vi "Get Named Tag Data.vi"(8 "error in (no error)":errorcluster, 10 "Tag Name":string, 11 "Raw Message in":refnum<class "Raw Message.lvclass">) -> (0 "error out":errorcluster, 1 "Tag Data":variant[](array[variant]), 2 "Key not found?":bool, 3 "Raw Message out":refnum<class "Raw Message.lvclass">)   [LabVIEW 2020]
uses:
  Raw Message.lvclass/Raw Message.ctl
  Tag/Basic Type.lvclass
  Raw Message.lvclass
  E:/Labview/LV 2020/Libs/LV Protobuf Raw/Source/Tag/Basic Type.lvclass
  E:/Labview/LV 2020/Libs/LV Protobuf Raw/Source/Proto Value/Proto Type.lvclass
  E:/Labview/LV 2020/Libs/LV Protobuf Raw/Source/Type Serializer/Type Serializer.lvclass
  E:/Labview/LV 2020/Libs/LV Protobuf Raw/Source/String Representable/String Representable.lvclass
  E:/Labview/LV 2020/Libs/LV Protobuf Raw/Source/Wire Type Group/Wire Type Group.lvclass
  E:/Labview/LV 2020/Libs/LV Protobuf Raw/Source/LEN Encoder/LEN.lvclass
  E:/Labview/LV 2020/Libs/LV Protobuf Raw/Source/Message/Raw Message.lvclass
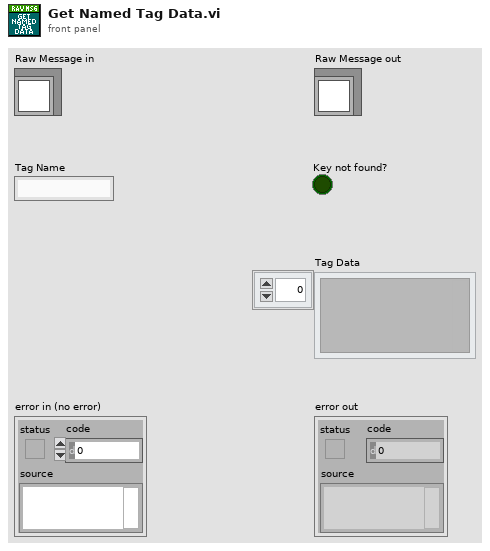
[diagram p1: front panel]
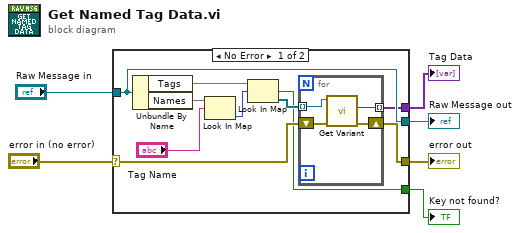
[diagram p0: block diagram]
diagram:
  n1 = case shown="No Error" "error in (no error)" {
    selector: "error in (no error)" -> [w15 w22]
    tunnel: [w14 w22] -> w5
    tunnel: [w16 w21] -> w3
    tunnel: "Raw Message in" -> [w16 w21]
    tunnel: [w10 _] -> w2
    tunnel: [w13 _] -> w1
    frame No Error {
      n2 = Unbundle By Name(w16) -> ("Tags"=w12, "Names"=w9)
      n3 = Look In Map(map=w9, key="Tag Name") -> (value=w7:u32)  [unwired: 1 in, 1 out]
      n4 = Look In Map(map=w12, key=w7) -> (key not found?=w10:bool, value=w11:refnum<class "Basic Type.lvclass">[])  [unwired: 1 in]
      n5 = for {
        tunnel: [w18] -> w13 mode=indexing
        tunnel: w11 -> [w17] mode=indexing
        shift-right: [w19] -> w14
        shift-left: w15 -> [w20]
        n6 = call-dynamic "Get Variant.vi"("error in (no error)"=w20, "Type Serializer in"=w17) -> ("error out"=w19:errorcluster, "Variant"=w18:variant)  [unwired: 7 in, 1 out]
      }
    }
    frame Error {
    }
  }
  "error out" <- w5
  "Raw Message out" <- w3
  "Key not found?" <- w2
  "Tag Data" <- w1
